vi "mgcVI HIGHLIGHT.vi"() -> ()   [LabVIEW 2018]
uses:
  <vilib>/Instr/_visa.llb/VISA Configure Serial Port (Instr).vi
panel:
  out "result string":string
  in  "stop 2":bool
  in  "VISA resource name":refnum<visa-resource-name>
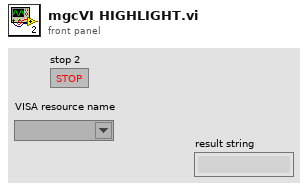
[diagram p1: front panel]
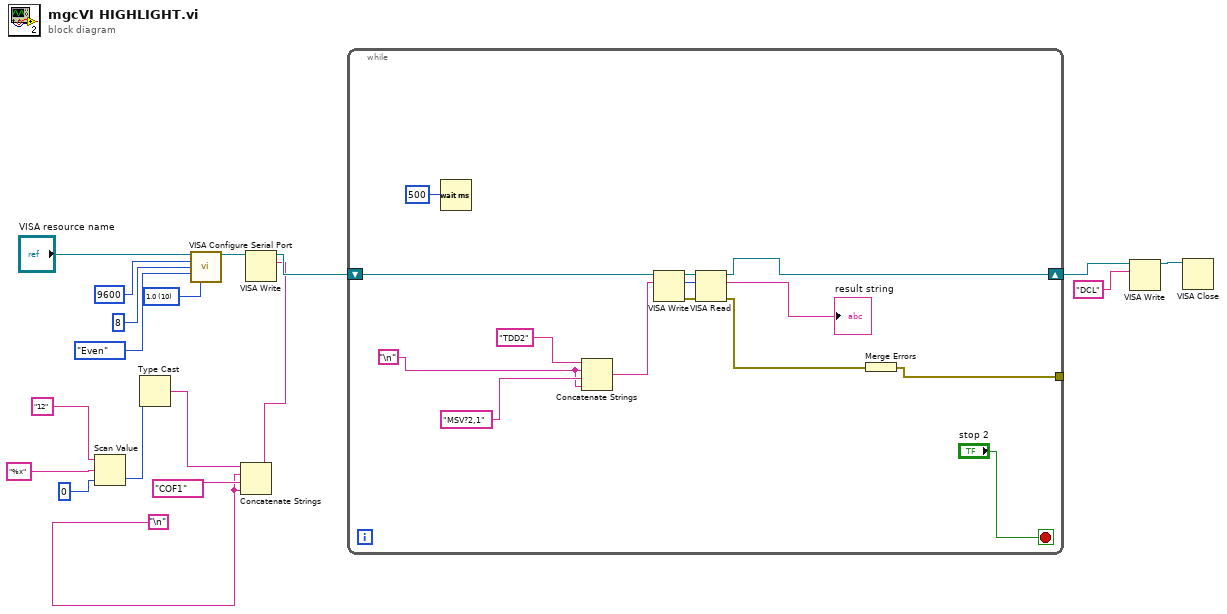
[diagram p0: block diagram]
diagram:
  w1 = "\n"
  w14 = u16 10 items=["1.0"=10, "1.5"=15, "2.0"=20] ("stop bits (10: 1 bit)")
  n1 = Scan Value(string="12", format string="%x", default (0 dbl)=0) -> (value=w9:i32)  [unwired: 1 out]
  n2 = Type Cast(x=w9) -> (*(type *) &x=w6:string)  [unwired: 1 in]
  n3 = call-poly "VISA Configure Serial Port"("VISA resource name"="VISA resource name", "baud rate (9600)"=u32 9600, "data bits (8)"=u16 8, "parity (0:none)"=enum16{"None", "Odd", "Even", "Mark", "Space"}."Even", "stop bits (10: 1 bit)"=w14) -> ("VISA resource name out"=w10:refnum<visa-resource-name>)  [unwired: 9 in, 1 out]
  n4 = Concatenate Strings(w6, w1, "COF1" ("Combo Box"), w1) -> (w7:string)
  n5 = VISA Write(VISA resource name=w10, write buffer=w7) -> (VISA resource name out=w8:refnum<visa-resource-name>)  [unwired: 1 in, 2 out]
  n6 = while {
    tunnel: [w24] -> _
    shift-right: [w21] -> w5
    shift-left: w8 -> [w25]
    stop <- "stop 2" stop-if-true
    w19 = "\n"
    n7 = Wait (ms)(milliseconds to wait=u32 500) -> ()  [unwired: 1 out]
    n8 = Concatenate Strings("TDD2" ("string"), w19, "MSV?2,1" ("write buffer"), w19) -> (w28:string)
    n9 = VISA Write(VISA resource name=w25, write buffer=w28) -> (VISA resource name out=w29:refnum<visa-resource-name>, return count=w31:u32, error out=w32:errorcluster)  [unwired: 1 in]
    n10 = VISA Read(VISA resource name=w29, byte count=w31, error in (no error)=w32) -> (VISA resource name out=w21:refnum<visa-resource-name>, read buffer=→"result string":string, error out=w30:errorcluster)  [unwired: 1 out]
    n11 = Merge Errors(w30) -> (w24:errorcluster)
  }
  n12 = VISA Write(VISA resource name=w5, write buffer="DCL") -> (VISA resource name out=w4:refnum<visa-resource-name>)  [unwired: 1 in, 2 out]
  n13 = VISA Close(VISA resource name=w4) -> ()  [unwired: 1 in, 1 out]
